vi "VISA Factory Wrapper.vi"(8 "error in (no error)":errorcluster, 10 "VISA settings":T1) -> (0 "error out":errorcluster, 3 "VISA out":refnum<class "VISA.lvclass">)   [LabVIEW 2018, in "Instrument Addon Scripting API.lvlib"]
doc: "Instantiates a new VISA Protocol object using the provided VISA settings."
uses:
  Instrument Addon Scripting API.lvlib
  Addon/Support Libraries/Protocols.lvlibp/VISA/VISA Settings.ctl
  Addon/Support Libraries/Protocols.lvlibp/VISA/VISA.lvclass
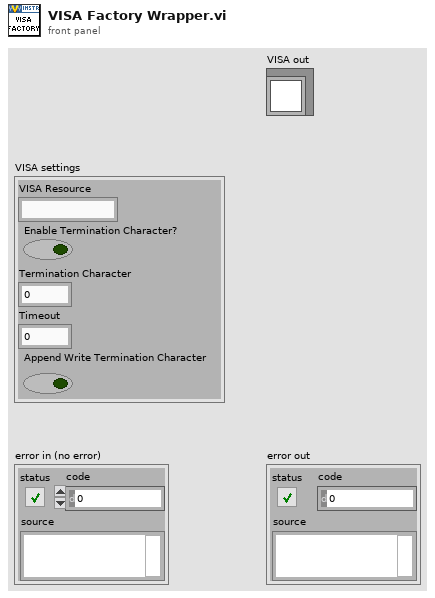
[diagram p1: front panel]
types:
  T1 = typedef "Protocols.lvlibp/VISA.lvclass/VISA Settings.ctl" = cluster{"VISA Resource":string, "Enable Termination Character?":bool, "Termination Character":u8, "Timeout":u32, "Append Write Termination Character":bool}
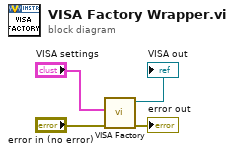
[diagram p0: block diagram]
diagram:
  n1 = call "VISA Factory.vi"("Error In"="error in (no error)", "VISA Settings"="VISA settings") -> ("Error Out"=→"error out":errorcluster, "VISA Out"=→"VISA out":refnum<class "VISA.lvclass">)  [unwired: 8 in]
